vi "Gripper.vi"() -> ()   [LabVIEW 2018]
uses:
  <vilib>/Rock Robotics/SystemInterfaces/DIO/FPGA_DIOPWMChannel.ctl
  <vilib>/Rock Robotics/SystemInterfaces/DIO/FPGA_DIOChannel.ctl
  <vilib>/ptbypt/NI_PtbyPt.lvlib
panel:
  in  "stop":bool
  in  "debug mode":bool
  in  "upper lim":dbl=0.52
  in  "lower lim":dbl=0.15 format="%#_13g"
  in  "toggle":bool
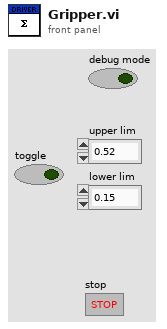
[diagram p1: front panel]
types:
  T1 = typedef "FPGA_DIOChannel.ctl" = enum8{"DIO 0", "DIO 1", "DIO 2", "DIO 3", "DIO 4", "DIO 5", "DIO 6", "DIO 7", "DIO 8", "DIO 9", "DIO MXP 0", "DIO MXP 1", "DIO MXP 2", "DIO MXP 3", "DIO MXP 4", "DIO MXP 5", "DIO MXP 6", "DIO MXP 7", "DIO MXP 8", "DIO MXP 9", "DIO MXP 10", "DIO MXP 11", "DIO MXP 12", "DIO MXP 13", "DIO MXP 14", "DIO MXP 15", "SPI Port CS1", "SPI Port CS2", "SPI Port CS3", "SPI Port MISO", "SPI Port MOSI", "Invalid"}
  T2 = typedef "FPGA_DIOPWMChannel.ctl" = enum8{"PWM 0", "PWM 1", "PWM 2", "PWM 3", "PWM 4", "PWM 5", "PWM 6", "PWM 7", "PWM 8", "PWM 9", "PWM MXP 0", "PWM MXP 1", "PWM MXP 2", "PWM MXP 3", "PWM MXP 4", "PWM MXP 5", "PWM MXP 6", "PWM MXP 7", "PWM MXP 8", "PWM MXP 9", "Invalid"}
  T3 = typedef "WPI_ServoDeviceRef.ctl" = cluster{"DeviceStatus":errorcluster, "PWM Channel":T2, "DeadBand":T4}
  T4 = typedef "WPI_PWMDeadband.ctl" = cluster{"Name":string, "maxPositivePwm":i32, "minPositivePwm":i32, "centerPwm":i32, "maxNegativePwm":i32, "minNegativePwm":i32, "angularRange":u16}
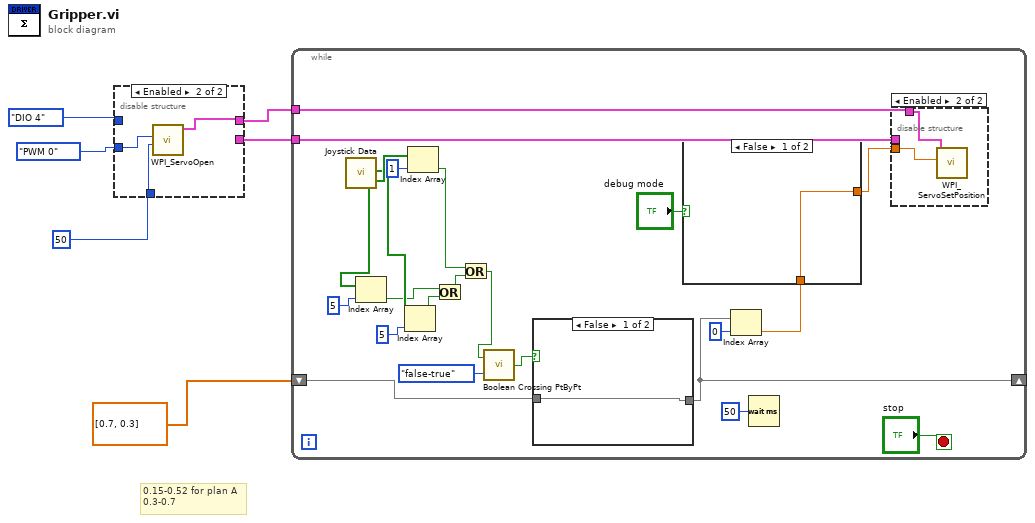
[diagram p0: block diagram]
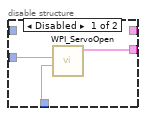
[diagram p2: hidden frame]
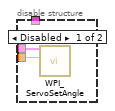
[diagram p3: hidden frame]
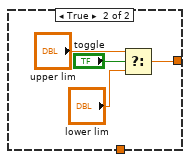
[diagram p4: hidden frame]
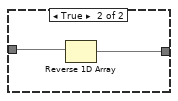
[diagram p5: hidden frame]
diagram:
  # "0.15-0.52 for plan A\n0.3-0.7"
  n1 = disable-structure shown="Enabled" {
    disable-tunnel: u16 50 ("Angular Range") -> [w9 w10]
    disable-tunnel: FPGA_DIOPWMChannel."PWM 0" ("PWM Channel") -> [w8 w11]
    disable-tunnel: [w7 _] -> w4
    disable-tunnel: FPGA_DIOChannel."DIO 4" ("DIO Channel") -> [_ _]
    disable-tunnel: [_ w12] -> w1
    frame Disabled {
      n2 = call <vilib>:"WPI_ServoOpen.vi"("Angular Range"=w9, "PWM Channel"=w8) -> ("ServoDeviceRef"=w7:T3)  [unwired: 8 in, 1 out]
    }
    frame Enabled {
      n3 = call <vilib>:"WPI_ServoOpen.vi"("Angular Range"=w10, "PWM Channel"=w11) -> ("ServoDeviceRef"=w12:T3)  [unwired: 8 in, 1 out]
    }
  }
  n4 = while {
    tunnel: w4 -> [w34]
    shift-right: [w30] -> _
    shift-left: dbl[] [0.7, 0.3] ("Array 2") -> [w28]
    tunnel: w1 -> [w19]
    stop <- "stop" stop-if-true
    n5 = call "Joystick Data.vi"() -> ("Controller Buttons Out"=w16:bool[], "Xbox Out"=w18:bool[], "Right Buttons Out"=w27:bool[])  [unwired: 13 in, 4 out]
    n6 = Index Array(array=w16, index=5) -> (element=w14:bool)
    n7 = Index Array(array=w18, index=5) -> (element=w15:bool)
    n8 = Index Array(array=w27, index=1) -> (element=w25:bool)
    n9 = Or(x=w14, y=w15) -> (x .or. y?=w13:bool)
    n10 = Or(x=w25, y=w13) -> (x .or. y?=w24:bool)
    n11 = call <vilib>:"Boolean Crossing PtByPt.vi"("direction"=enum16{"either", "false-true", "true-false"}."false-true", "input"=w24) -> ("crossing"=w31:bool)  [unwired: 1 in]
    n12 = case shown="False" w31 {
      tunnel: [w45 w47] -> w30
      tunnel: w28 -> [w45 w46]
      frame False {
      }
      frame True {
        n13 = Reverse 1D Array(array=w46) -> (reversed array=w47:dbl[])
      }
    }
    n14 = Index Array(array=w30, index=0) -> (element=w21:dbl)
    n15 = case shown="False" "debug mode" {
      tunnel: [w40 w41] -> w23
      tunnel: w21 -> [w40 _]
      frame False {
      }
      frame True {
        n16 = Select(t="upper lim", s="toggle", f="lower lim") -> (s? t:f=w41:dbl)
      }
    }
    n17 = Wait (ms)(milliseconds to wait=u32 50) -> ()  [unwired: 1 out]
    n18 = disable-structure shown="Enabled" {
      disable-tunnel: w34 -> [w37 _]
      disable-tunnel: w23 -> [w36 w39]
      disable-tunnel: w19 -> [_ w38]
      frame Disabled {
        n19 = call <vilib>:"WPI_ServoSetAngle.vi"("Angle"=w36, "ServoDeviceRef"=w37) -> ()  [unwired: 8 in, 2 out]
      }
      frame Enabled {
        n20 = call <vilib>:"WPI_ServoSetPosition.vi"("Position"=w39, "ServoDeviceRef"=w38) -> ()  [unwired: 8 in, 2 out]
      }
    }
  }
